vi "Pre Launch Init.vi"(11 "WebServer in":refnum<class "MonSys_Server_Actor.lvclass">) -> (0 "error out":errorcluster, 3 "WebServer out":refnum<class "MonSys_Server_Actor.lvclass">)   [LabVIEW 2018, in "MonSys_Server_Actor.lvlib" / "MonSys_Server_Actor.lvclass"]
doc: "(<B>Filename</B>: Actor Framework.lvlib:Actor.lvclass:Pre Launch Init.vi)\n\nDefines behavior that occurs after the Launch Nested Actor method is invoked but before the actor's Actor Core method begins running.\n\nBy default, this method does nothing. A descendant class may override it to define behavior."
uses:
  MonSys_Server_Actor.lvclass
  typedefs/OnlineData_HandleDVR_func.ctl
  MonSys_Server_Actor.lvclass/MonSys_Server_Actor.ctl
  <vilib>/ActorFramework/Actor/Actor.lvclass
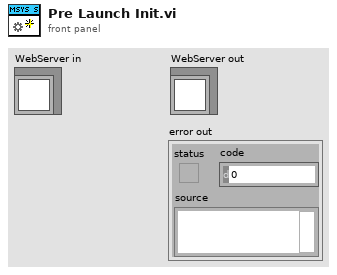
[diagram p1: front panel]
types:
  T1 = typedef "OnlineData_HandleDVR_func.ctl" = enum16{"create", "get", "close"}
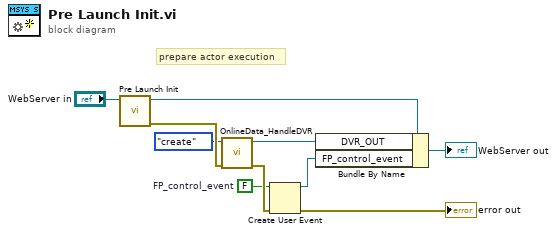
[diagram p0: block diagram]
diagram:
  w1 = FALSE  # FP_control_event
  # "prepare actor execution"
  n1 = call-parent "Pre Launch Init.vi"("Actor in"="WebServer in") -> ("error out"=w9:errorcluster, "Actor out"=w7:refnum<class "MonSys_Server_Actor.lvclass">)  [unwired: 9 in]
  n2 = call "OnlineData_HandleDVR.vi"("error in"=w9, "func"=OnlineData_HandleDVR_func."create") -> ("error out"=w4:errorcluster, "DVR_OUT"=w5:refnum<data-value>)  [unwired: 8 in]
  n3 = Create User Event(user event datatype=w1, error in=w4) -> (user event=w2:refnum<user-event>, error out=→"error out":errorcluster)
  n4 = Bundle By Name(cluster=w7, "DVR_OUT"=w5, "FP_control_event"=w2) -> (→"WebServer out":refnum<class "MonSys_Server_Actor.lvclass">)
